vi "FTW-CodeGen-Bounds.vi"(0 "State In":T1 {"Width" format="%dpx"}, 5 "XRef":refnum<vi>) -> (4 "Bounds":cluster{"Width":i32, "Height":i32})   [LabVIEW 2015, in "FTW-Dataflow-Burrow.xnode"]
uses:
  FTW-Dataflow-Burrow.xnode
  FTW-CodeGen-State.ctl
panel:
  # "Inputs"
  # "Outputs"
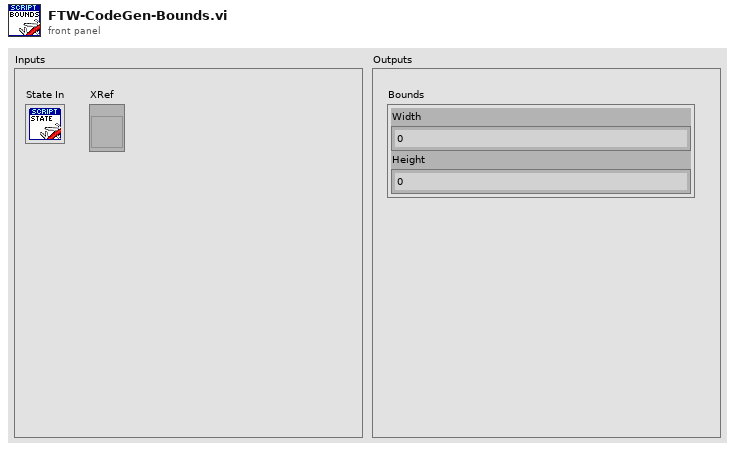
[diagram p1: front panel]
types:
  T1 = typedef "FTW-Dataflow-Burrow.xnode/FTW-CodeGen-State.ctl" = cluster{"InputTerminals":cluster{"Wired?":bool, "ID":string, "DataName":string, "DataColor":u32, "Type":variant}[], "EnableTiming?":bool, "Width":i32}
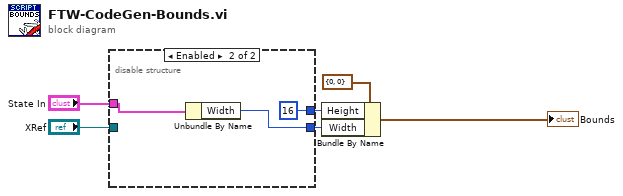
[diagram p0: block diagram]
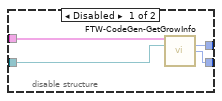
[diagram p2: hidden frame]
diagram:
  n1 = disable-structure shown="Enabled" {
    disable-tunnel: "State In" -> [w10 w13]
    disable-tunnel: "XRef" -> [w9 _]
    disable-tunnel: [w8 w11] -> w2
    disable-tunnel: [w7 16 ("Current Height")] -> w1
    frame Disabled {
      n2 = call "FTW-CodeGen-GetGrowInfo.vi"("State In"=w10, "XRef"=w9) -> ("Current Height"=w7:i32, "Width"=w8:i32)  [unwired: 5 in, 7 out]
    }
    frame Enabled {
      n3 = Unbundle By Name(w13) -> ("Width"=w11:i32)
    }
  }
  n4 = Bundle By Name(cluster=cluster{"Width":i32, "Height":i32} {"Width"=0, "Height"=0} ("Bounds"), "Height"=w1, "Width"=w2) -> (→"Bounds":cluster{"Width":i32, "Height":i32})
